vi "Example Graph.vi"() -> ()   [LabVIEW 2013]
uses:
  C:/tf/play/labview/Tinkerforge.dll
  Tinkerforge.dll
panel:
  in  "stop":bool
  out "graph":i32[](graph)
  in  "uid":string="amb"
  in  "port":i32=4223
  in  "host":string="localhost"
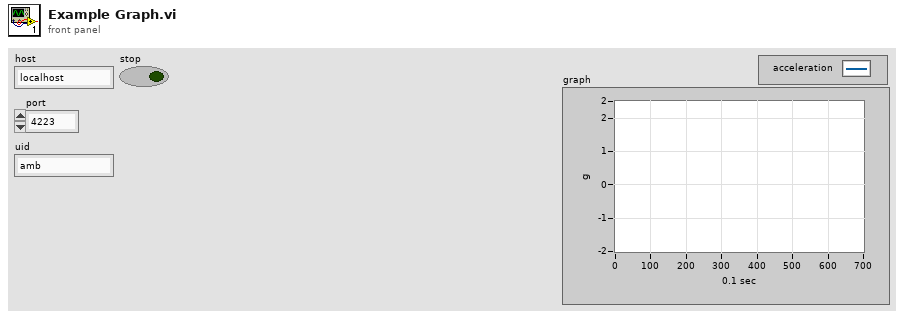
[diagram p1: front panel]
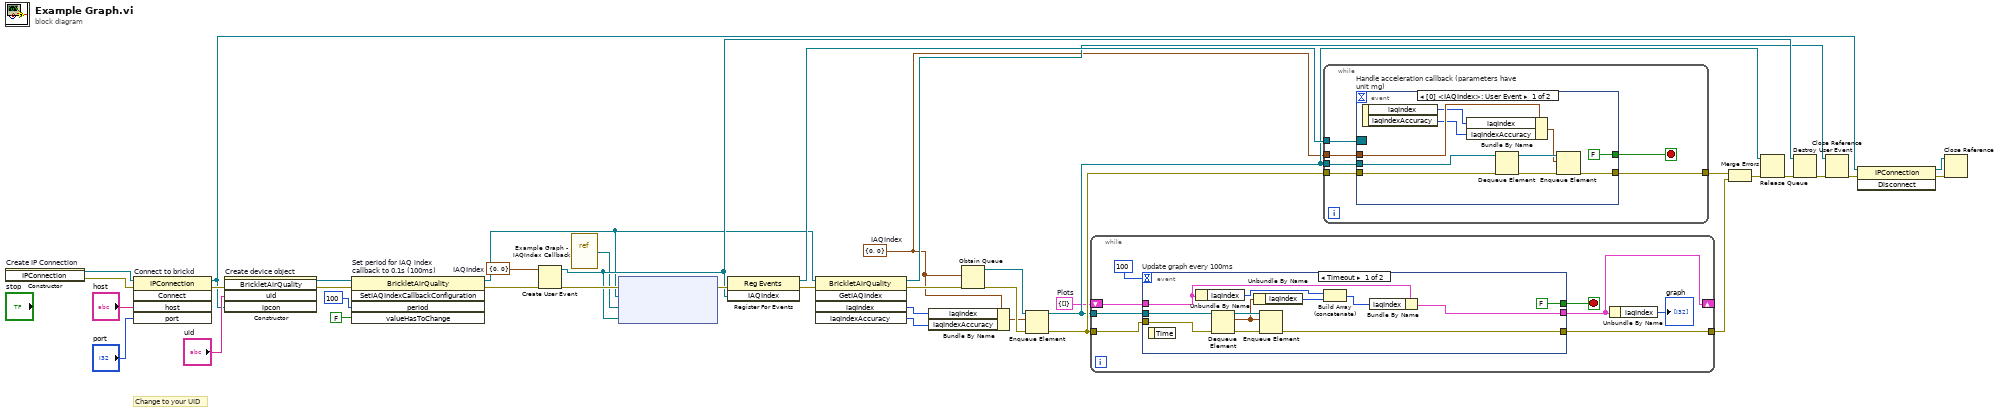
[diagram p0: block diagram]
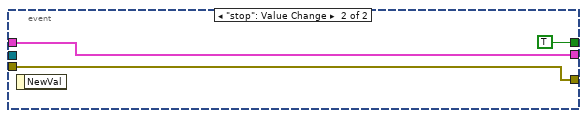
[diagram p2: hidden frame]
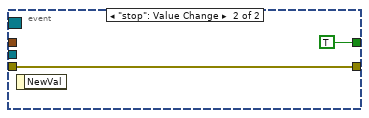
[diagram p3: hidden frame]
diagram:
  w3 = cluster{"iaqIndex":i32, "iaqIndexAccuracy":u8} {"iaqIndex"=0, "iaqIndexAccuracy"=0}  # IAQIndex
  w6 = cluster{"iaqIndex":i32[]} {"iaqIndex"=[]}  # Plots
  w25 = cluster{"iaqIndex":i32, "iaqIndexAccuracy":u8} {"iaqIndex"=0, "iaqIndexAccuracy"=0}  # IAQIndex
  # "Change to your UID"
  n1 = constructor on="Create IP Connection" class="IPConnection"() -> (reference out=w39:refnum<k24>, error out=w12:errorcluster)  [unwired: 3 in, 1 out]
  n2 = invoke on="Connect to brickd" class="IPConnection" method="Connect"(reference=w39, error in=w12, "host"="host", "port"="port") -> (reference out=w32:refnum<k24>, error out=w35:errorcluster)  [unwired: 1 in, 3 out]
  n3 = constructor on="Create device object" class="BrickletAirQuality"(error in=w35, "uid"="uid", "ipcon"=w32) -> (reference out=w22:refnum<k24>, error out=w24:errorcluster)  [unwired: 2 in, 3 out]
  n4 = invoke on="Set period for IAQ index\ncallback to 0.1s (100ms)" class="BrickletAirQuality" method="SetIAQIndexCallbackConfiguration"(reference=w22, error in=w24, "period"=i64 100, "valueHasToChange"=FALSE) -> (reference out=w9:refnum<k24>, error out=w23:errorcluster)  [unwired: 1 in, 3 out]
  n5 = Create User Event(user event datatype=w25, error in=w23) -> (user event=w27:refnum<user-event>, error out=w30:errorcluster)
  n6 = vi-ref "Example Graph - IAQIndex Callback.vi"() -> ("vi reference"=w1:refnum<vi>)
  n7 = node ("Register Event Callback")(w30, w9, w1, w27) -> (w29:errorcluster)  [unwired: 1 in, 1 out]
  n8 = register-events(error in=w29, w27) -> (reference out=w28:refnum<event-registration>, error out=w11:errorcluster)  [unwired: 1 in]
  n9 = invoke class="BrickletAirQuality" method="GetIAQIndex"(reference=w9, error in=w11) -> (reference out=w8:refnum<k24>, error out=w10:errorcluster, "iaqIndex"=w4:i32, "iaqIndexAccuracy"=w2:u8)  [unwired: 3 in, 1 out]
  n10 = Bundle By Name(cluster=w3, "iaqIndex"=w4, "iaqIndexAccuracy"=w2) -> (w7:cluster{"iaqIndex":i32, "iaqIndexAccuracy":u8})
  n11 = Obtain Queue(element data type=w3, error in (no error)=w10) -> (queue out=w16:refnum<queue>, error out=w18:errorcluster)  [unwired: 3 in, 1 out]
  n12 = Enqueue Element(queue=w16, element=w7, error in (no error)=w18) -> (queue out=w13:refnum<queue>, error out=w17:errorcluster)  [unwired: 1 in, 1 out]
  n13 = while {
    tunnel: [w44] -> w20
    tunnel: w17 -> [w45]
    shift-right: [w41] -> _
    shift-left: w6 -> [w46]
    tunnel: w13 -> [w43]
    stop <- w42 stop-if-true
    n14 = event "Update graph every 100ms" shown="[0] Timeout" {
      selector: _ -> [_ _]
      dyn-events: _ -> [_ _]
      timeout: 100 -> [_ _]
      tunnel: [w51 w61] -> w41
      tunnel: w46 -> [w52 w61]
      tunnel: w45 -> [w59 w60]
      tunnel: [w56 w60] -> w44
      tunnel: w43 -> [w58 _]
      tunnel: [FALSE TRUE] -> w42
      event Timeout {
        n15 = event-data() -> ()  [unwired: 1 in, 1 out]
        n16 = Unbundle By Name(w52) -> ("iaqIndex"=w50:i32[])
        n17 = Dequeue Element(queue=w58, error in (no error)=w59) -> (queue out=w55:refnum<queue>, element=w53:cluster{"iaqIndex":i32, "iaqIndexAccuracy":u8}, error out=w57:errorcluster)  [unwired: 1 in, 1 out]
        n18 = Unbundle By Name(w53) -> ("iaqIndex"=w48:i32)
        n19 = Enqueue Element(queue=w55, element=w53, error in (no error)=w57) -> (error out=w56:errorcluster)  [unwired: 1 in, 2 out]
        n20 = Build Array (concatenate)(w50, w48) -> (w49:i32[])
        n21 = Bundle By Name(cluster=w52, "iaqIndex"=w49) -> (w51:cluster{"iaqIndex":i32[]})
      }
      event "stop": Value Change {
        n22 = event-data() -> ()  [unwired: 1 in, 1 out]
      }
    }
    n23 = Unbundle By Name(w41) -> ("iaqIndex"=→"graph":i32[])
  }
  n24 = while {
    tunnel: w28 -> [w68]
    tunnel: [w66] -> w19
    tunnel: w17 -> [w67]
    tunnel: w13 -> [w65]
    tunnel: w3 -> [w63]
    stop <- w64 stop-if-true
    n25 = event "Handle acceleration callback (parameters have unit mg)" shown="[0] <IAQIndex>: User Event" {
      selector: w68 -> [_ _]
      dyn-events: _ -> [_ _]
      timeout: _ -> [_ _]
      tunnel: w67 -> [w78 w79]
      tunnel: [w76 w79] -> w66
      tunnel: w65 -> [w75 _]
      tunnel: [FALSE TRUE] -> w64
      tunnel: w63 -> [w71 _]
      event User Event {
        n26 = event-data() -> ("iaqIndex"=w70:i32, "iaqIndexAccuracy"=w69:u8)  [unwired: 1 in]
        n27 = Bundle By Name(cluster=w71, "iaqIndex"=w70, "iaqIndexAccuracy"=w69) -> (w72:cluster{"iaqIndex":i32, "iaqIndexAccuracy":u8})
        n28 = Dequeue Element(queue=w75, error in (no error)=w78) -> (queue out=w74:refnum<queue>, error out=w77:errorcluster)  [unwired: 1 in, 2 out]
        n29 = Enqueue Element(queue=w74, element=w72, error in (no error)=w77) -> (error out=w76:errorcluster)  [unwired: 1 in, 2 out]
      }
      event "stop": Value Change {
        n30 = event-data() -> ()  [unwired: 1 in, 1 out]
      }
    }
  }
  n31 = Merge Errors(w19, w20) -> (w15:errorcluster)
  n32 = Release Queue(queue=w13, error in (no error)=w15) -> (error out=w14:errorcluster)  [unwired: 1 in, 2 out]
  n33 = Destroy User Event(user event=w27, error in=w14) -> (error out=w26:errorcluster)
  n34 = Close Reference(reference=w8, error in (no error)=w26) -> (error out=w34:errorcluster)
  n35 = invoke class="IPConnection" method="Disconnect"(reference=w32, error in=w34) -> (reference out=w31:refnum<k24>, error out=w33:errorcluster)  [unwired: 1 in, 1 out]
  n36 = Close Reference(reference=w31, error in (no error)=w33) -> ()  [unwired: 1 out]
